vi "Stop Core.vi"(10 "final error code":i32, 11 "Alpha UI in":refnum<class "Simulated Wash Display Console.lvclass">) -> (3 "Alpha UI out":refnum<class "Simulated Wash Display Console.lvclass">)   [LabVIEW 2012, in "Simulated Wash Display Console.lvlib" / "Simulated Wash Display Console.lvclass"]
doc: "(<B>Filename</B>: Actor Framework.lvlib:Actor.lvclass:Stop Core.vi)\n\nDefines what the actor does before it stops. Use the <B>final error code</B> input to determine whether the actor shut down in response to an error.\n\nBy default, this method does nothing. A descendant class may override it to define behavior, such as shutting down any processes the actor initiated in its override of the Actor Core method."
uses:
  Simulated Wash Display Console/Simulated Wash Display Console.lvclass
  Wash Display Console API/Wash Display Console API/Wash Display Console API.lvclass
  Simulated Wash Display Console/Simulated Wash Display Console.lvclass/Simulated Wash Display Console.ctl
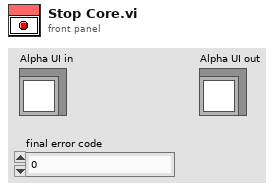
[diagram p1: front panel]
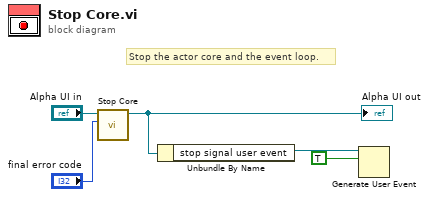
[diagram p0: block diagram]
diagram:
  # "Stop the actor core and the event loop."
  n1 = call-parent "Stop Core.vi"("final error code"="final error code", "Actor in"="Alpha UI in") -> ("Actor out"=w3:refnum<class "Simulated Wash Display Console.lvclass">)  [unwired: 9 in]
  "Alpha UI out" <- w3
  n2 = Unbundle By Name(w3) -> ("stop signal user event"=w2:refnum<user-event>)
  n3 = Generate User Event(user event=w2, event data cluster=TRUE ("event data")) -> ()  [unwired: 1 in, 2 out]
